vi "2 Tap 10-8-Bit.vi"() -> (0 "PixelData":cluster{"Pixel 0":u16, "Pixel 1":u16})   [LabVIEW 2016]
uses:
  <vilib>/rvi/eio/common/nirviEmuTemplateMethod_errors.vi
  <vilib>/eio/EIONode/EIONode.xnode
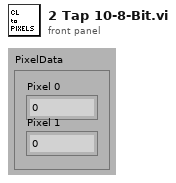
[diagram p1: front panel]
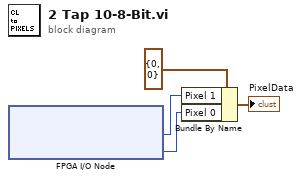
[diagram p0: block diagram]
diagram:
  n1 = xnode "FPGA I/O Node"() -> ("IO Module\\CL Port C"=w1:u8, "IO Module\\CL Port A"=w2:u8)  [unwired: 2 in, 2 out]
  n2 = Bundle By Name(cluster=cluster{"Pixel 0":u16, "Pixel 1":u16} {"Pixel 0"=0, "Pixel 1"=0} ("PixelData"), "Pixel 1"=w1, "Pixel 0"=w2) -> (→"PixelData":cluster{"Pixel 0":u16, "Pixel 1":u16})
